vi "xy graph from 1d arrays.vi"(1 "y2":dbl[](array[numeric]), 2 "y1":dbl[](array[numeric]), 3 "shot#":i32, 4 "x":dbl[](array[numeric])) -> (0 "xy graph":cluster{"Ramp Pattern":dbl[], dbl[]}[](array[cluster]))   [LabVIEW 2013]
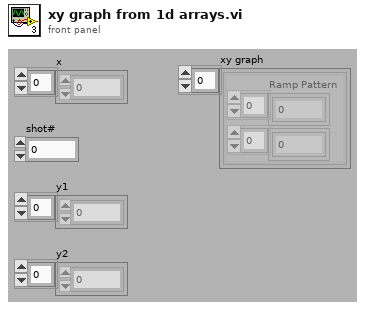
[diagram p1: front panel]
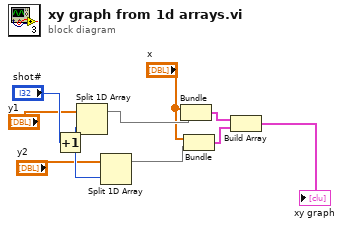
[diagram p0: block diagram]
diagram:
  n1 = Increment(x="shot#") -> (x+1=w9:i32)
  n2 = Split 1D Array(array="y1", index=w9) -> (first subarray=w6:dbl[])  [unwired: 1 out]
  n3 = Split 1D Array(array="y2", index=w9) -> (first subarray=w10:dbl[])  [unwired: 1 out]
  n4 = Bundle("x"="x", w6) -> (w2:cluster{"x":dbl[], dbl[]})  [unwired: 1 in]
  n5 = Bundle("x"="x", w10) -> (w1:cluster{"x":dbl[], dbl[]})  [unwired: 1 in]
  n6 = Build Array(w2, w1) -> (→"xy graph":cluster{"x":dbl[], dbl[]}[])
